vi "Global.vi"() -> ()   [LabVIEW 2024]
panel:
  in  "Station 3 IP ADDRESS":string="192.168.3.250"
  in  "Station 2 IP ADDRESS":string="192.168.3.252"
  in  "Station 1 IP ADDRESS":string="192.168.3.254"
  in  "emg":bool
  out "Command":string="*IDN?\n"
  in  "Exit":bool
  # "2*192.168.3.254: op 10"
  # "192.168.3.252: op 30"
  # "192.168.3.250 : op 40"
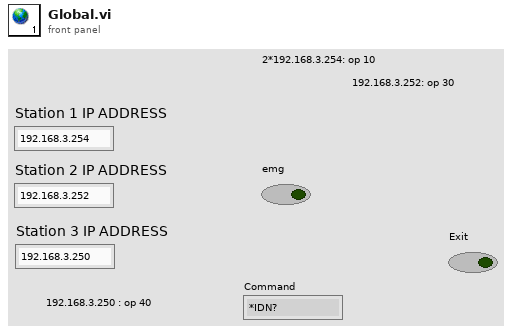
[diagram p1: front panel]
diagram:
